vi "Add Transfer Group with Children.vi"(6 "Plugin Decimation (1)":u64=1, 8 "error in (no error)":errorcluster, 9 "Transfer Group":refnum<class "Transfer Group.lvclass">, 10 "parent tag":string, 11 "Application Data In":T1) -> (0 "error out":errorcluster, 3 "Application Data In":T1)   [LabVIEW 2017, in "DSF Data Viewer.lvlib"]
uses:
  DSF Data Viewer.lvlib
  Main VI/Application Data.ctl
  Builds/Data Sharing Framework/Current/Core/DSF Core.lvlibp/Engine/Classes/Framework/Framework.lvclass
  <vilib>/NI/Memory Manager/Classes/Pointer/Pointer.lvclass
  Buffer Reader/Buffer Data.ctl
  Builds/Data Sharing Framework/Current/Core/DSF Core.lvlibp/Engine/Classes/Buffer/Buffer.lvclass
  Builds/Data Sharing Framework/Current/Core/DSF Core.lvlibp/Engine/Classes/Transfer Group/Transfer Group.lvclass
  ID to Tree Items/Tree Item Type.ctl
  Add Buffers.vi
  Builds/Data Sharing Framework/Current/Core/DSF Core.lvlibp/Engine/Classes/Buffer/Get String Buffer.vi
  Builds/Data Sharing Framework/Current/Core/DSF Core.lvlibp/Engine/Classes/Buffer/Get Async Buffer.vi
  Builds/Data Sharing Framework/Current/Core/DSF Core.lvlibp/Engine/Classes/Buffer/Get Inline Buffer.vi
  Builds/Data Sharing Framework/Current/Core/DSF Core.lvlibp/Engine/Classes/Transfer/Get Buffers.vi
  Builds/Data Sharing Framework/Current/Core/DSF Core.lvlibp/Engine/Classes/Timing/Timing.lvclass
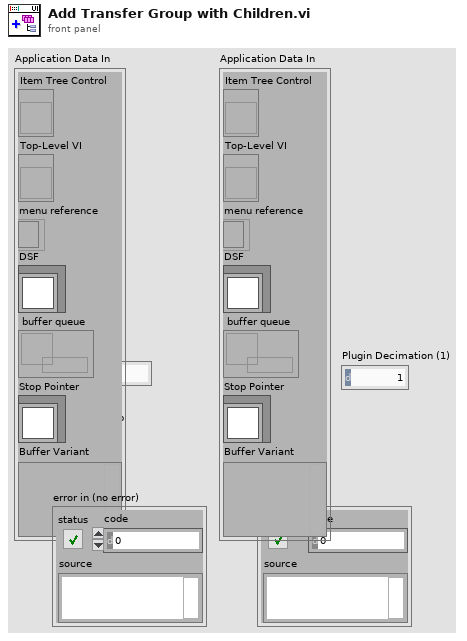
[diagram p1: front panel]
types:
  T1 = typedef "DSF Data Viewer.lvlib/Application Data.ctl" = cluster{"Item Tree Control":refnum<vi>, "Top-Level VI":refnum<vi>, "menu reference":refnum<k9>, "DSF":refnum<class "Framework.lvclass">, "buffer queue":refnum<queue>, "Stop Pointer":refnum<class "Pointer.lvclass">, "Buffer Variant":variant}
  T2 = typedef "DSF Data Viewer.lvlib/Buffer Data.ctl" = cluster{"Buffer":refnum<class "Buffer.lvclass">, "decimation":u64}
  T3 = typedef "DSF Data Viewer.lvlib/Tree Item Type.ctl" = enum16{"Framework", "Plugin Group", "Plugin", "Group", "Transfer", "Buffer", "Channel"}
  T4 = typedef "DSF Data Viewer.lvlib/Tree Item.ctl" = cluster{"Left Cell String":string, "Child Text":string[], "Child Tag":string, "Glyph Index":i32}
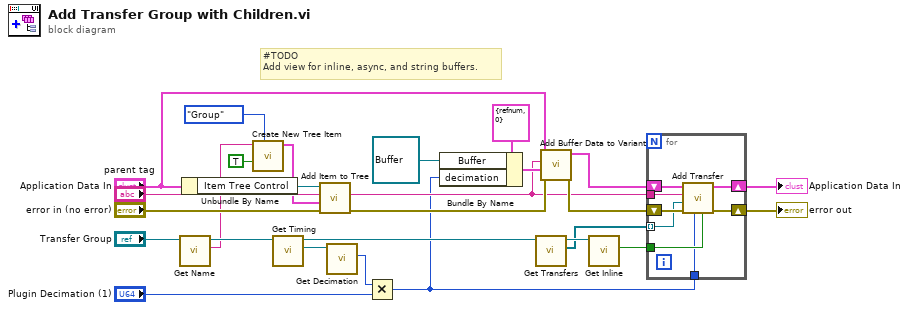
[diagram p0: block diagram]
diagram:
  # "#TODO\nAdd view for inline, async, and string buffers."
  n1 = call "Get Name.vi"("Transfer Group in"="Transfer Group") -> ("name"=w1:string, "Transfer Group out"=w8:refnum<class "Transfer Group.lvclass">)  [unwired: 9 in]
  n2 = Unbundle By Name("Application Data In") -> ("Item Tree Control"=w16:refnum<vi>)
  n3 = call "Create New Tree Item.vi"("Item Type"=Tree_Item_Type."Group", "found?"=TRUE, "Left Cell String"=w1) -> ("Item"=w22:T4)  [unwired: 7 in, 1 out]
  n4 = call "Get Timing.vi"("Transfer Group in"=w8) -> ("Timing"=w6:refnum<class "Timing.lvclass">, "Transfer Group out"=w7:refnum<class "Transfer Group.lvclass">)  [unwired: 9 in]
  n5 = call "Add Item to Tree.vi"("error in (no error)"="error in (no error)", "Item"=w22, "parent tag"="parent tag", "TreeControl in"=w16) -> ("error out"=w11:errorcluster, "new item tag"=w3:string)  [unwired: 5 in, 1 out]
  n6 = call "Get Decimation.vi"("Timing in"=w6) -> ("Decimation"=w5:u64)  [unwired: 9 in, 1 out]
  n7 = Multiply(x=w5, y="Plugin Decimation (1)") -> (x*y=w2:u64)
  n8 = Bundle By Name(cluster=T2 {"Buffer"=refnum, "decimation"=0} ("Buffer data"), "Buffer"=refnum<class "Buffer.lvclass"> refnum, "decimation"=w2) -> (w14:T2)
  n9 = call "Get Transfers.vi"("Transfer Group in"=w7) -> ("Transfers"=w19:refnum<class "Transfer.lvclass">[], "Transfer Group out"=w21:refnum<class "Transfer Group.lvclass">)  [unwired: 9 in]
  n10 = call "Add Buffer Data to Variant.vi"("error in (no error)"=w11, "Buffer data"=w14, "tag"=w3, "Application Data In in"="Application Data In") -> ("error out"=w10:errorcluster, "Application Data In out"=w12:T1)  [unwired: 6 in]
  n11 = call "Get Inline.vi"("Transfer Group in"=w21) -> ("inline"=w20:bool)  [unwired: 9 in, 1 out]
  n12 = for {
    shift-right: [w33] -> w18
    shift-left: w12 -> [w35]
    shift-right: [w32] -> w17
    shift-left: w10 -> [w34]
    tunnel: w19 -> [w31] mode=indexing
    tunnel: w3 -> [w30]
    tunnel: w20 -> [w29]
    tunnel: w2 -> [w28]
    n13 = call "Add Transfer.vi"("inline"=w29, "Group Decimation (1)"=w28, "error in (no error)"=w34, "Transfer"=w31, "parent tag"=w30, "Application Data In"=w35) -> ("error out"=w32:errorcluster, "Application Data Out"=w33:T1)  [unwired: 4 in]
  }
  "error out" <- w17
  "Application Data In" <- w18
